vi "medicaoIXV.vi"() -> ()   [LabVIEW 2012]
uses:
  <vilib>/Utility/file.llb/Write To Spreadsheet File (string).vi
  <vilib>/Utility/file.llb/Write To Spreadsheet File (DBL).vi
  <instrlib>/Agilent 6XXX Series/Agilent 6XXX Series.lvlib
panel:
  out "reset graph":bool=TRUE
  out "tabela":dbl[][](array[numeric])
  in  "Tab Control":enum32{"Entrada de dados", "Saída de dados"}(tab)
  in  "T.J":dbl caption="Tensão\ndo joelho"
  in  "p.a.j":dbl caption="Pontos antes\ndo joelho"
  in  "nMedições":i16=1 caption="N° medições" min=1
  in  "area":dbl caption="Área da célula"
  in  "Tipo":string caption="Tipo da célula"
  in  "Formato":u16(ring) items=[".txt", ".csv"]
  out "ON/OFF1":bool caption="ON/OFF"
  in  "p.d.j":dbl caption="Pontos depois\ndo joelho"
  in  "T.M":dbl caption="Tensão máxima"
  in  "Nome da célula":string
  in  "Local":path
  in  "Delay(ms)":dbl
  in  "Start":bool
  in  "temperatura":dbl caption="Temperatura da célula"
  in  "stopProgram":bool caption="Parar Programa"
  out "Imp":dbl
  out "Vmp":dbl
  out "Pmp":dbl
  out "Icc (A)":dbl
  out "Vca (V)":dbl
  in  "Print Screen":bool
  out "IXV":cluster{"Y":dbl[], "Y":dbl[]}[](graph)
  out "output voltage":dbl
  out "vAtual":dbl caption="Tensao Atual (V)"
  out "aAtual":dbl caption="Corrente Atual\n(A)"
  out "Ponto Atual":i32
  out "tabela":dbl[][](array[numeric]) caption="TABELA DE DADOS\nTensão(Fonte)      Pontos             Tensao           Corrente" format="%0.8f"
  in  "stop":bool caption="Parar Medição"
  out "ON/OFF2":bool caption="ON/OFF"
  in  "CorrenteGraph":dbl
  in  "TensaoGraph":dbl
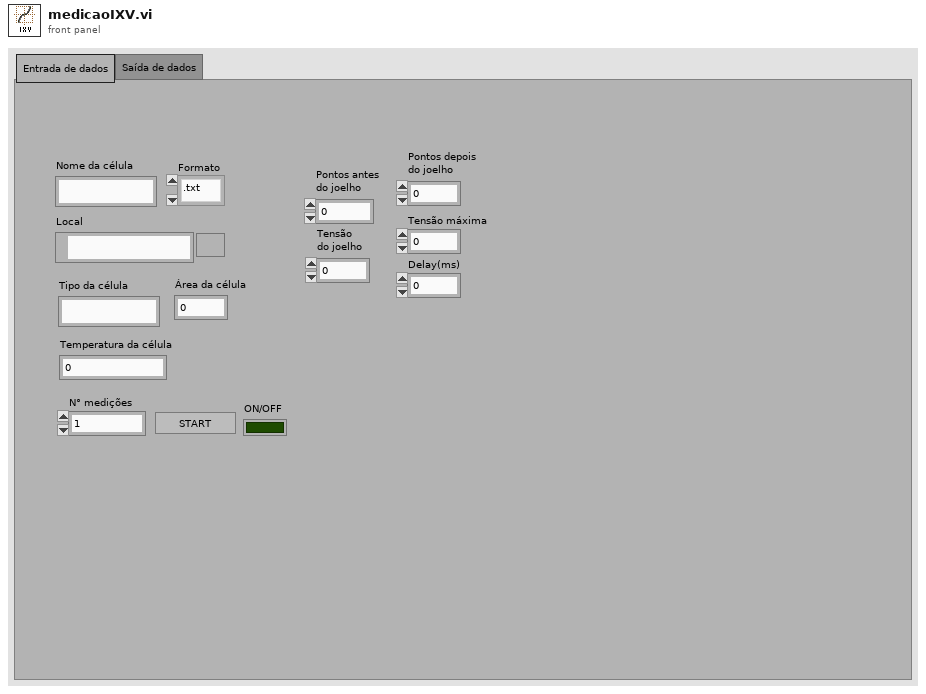
[diagram p1: front panel]
types:
  T1 = typedef "imagedata.ctl" = cluster{"image type":i32, "image depth":i32, "image":u8[], "mask":u8[], "colors":u32[], "Rectangle":cluster{"left":i16, "top":i16, "right":i16, "bottom":i16}}
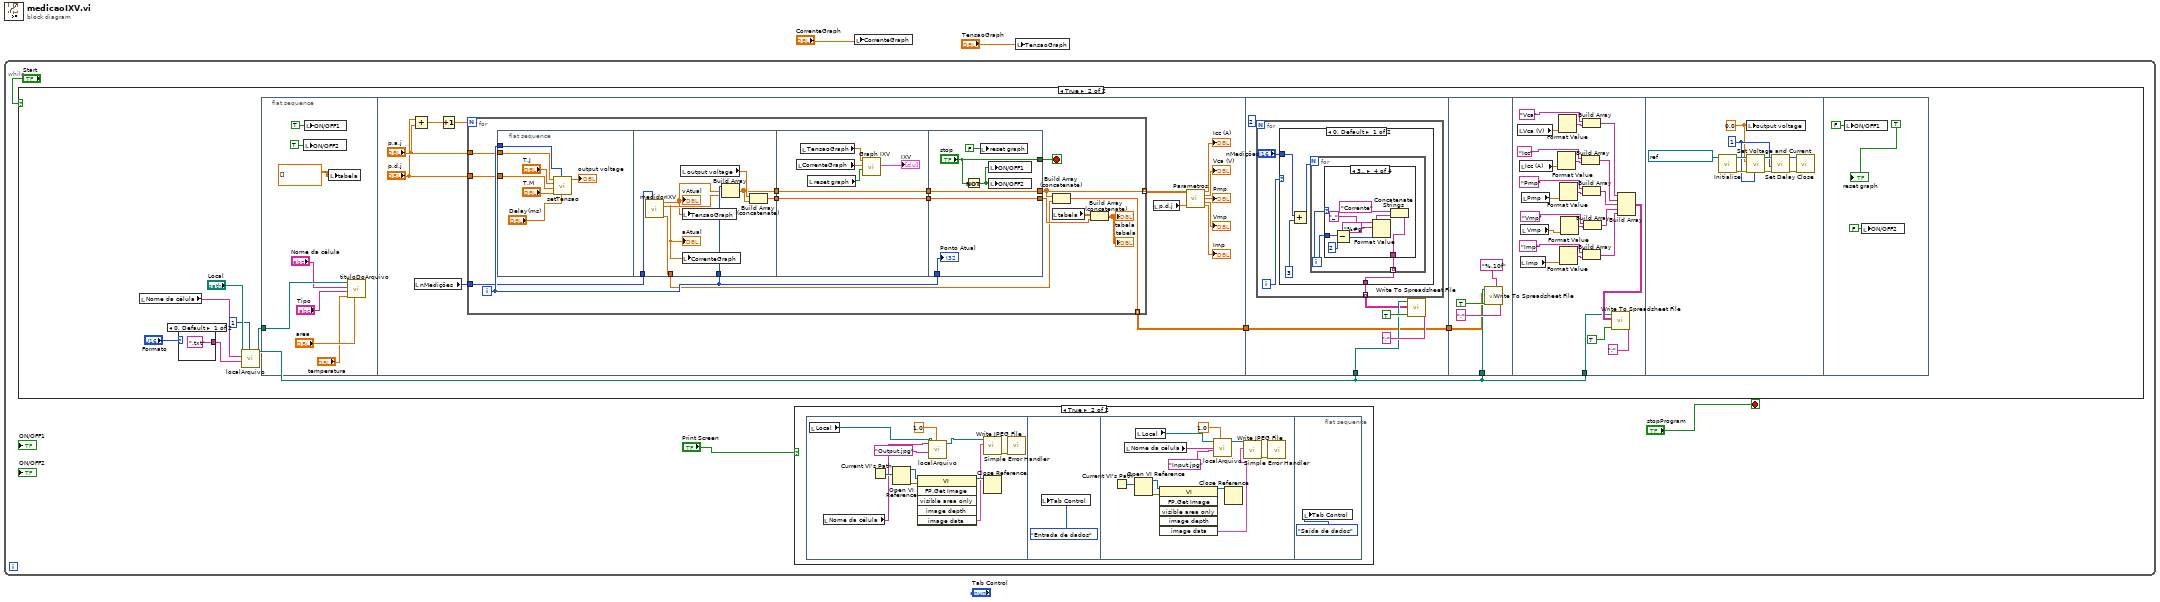
[diagram p0: block diagram]
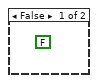
[diagram p3: hidden frame]
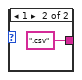
[diagram p4: hidden frame]
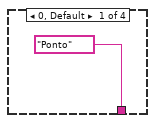
[diagram p5: hidden frame]
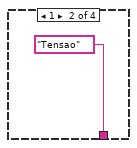
[diagram p6: hidden frame]
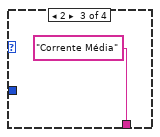
[diagram p7: hidden frame]
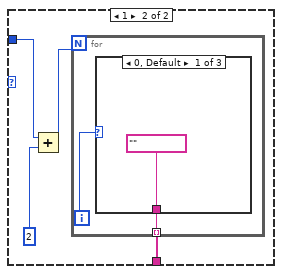
[diagram p8: hidden frame]
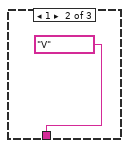
[diagram p9: hidden frame]
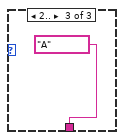
[diagram p10: hidden frame]
diagram:
  n1 = while {
    stop <- "stopProgram" stop-if-true
    n2 = case shown="True" "Start" {
      frame False {
        (unwired) FALSE
      }
      frame True {
        n3 = local read "Nome da célula"() -> (w35:string)
        n4 = case shown="0, Default" "Formato" {
          tunnel: [".txt" ".csv"] -> w34
          frame 0, Default {
          }
          frame 1 {
          }
        }
        n5 = call "localArquivo.vi"("quantidadeDeArquivos"=i16 1, "extensão"=w34, "Nome do arquivo"=w35, "Local"="Local") -> ("Path"=w33:path)  [unwired: 7 in]
        n6 = flat-sequence {
          tunnel: w33 -> [w47]
          tunnel: [w48] -> w30
          tunnel: w33 -> [w106]
          tunnel: [w103] -> w31
          tunnel: w30 -> [w103]
          tunnel: w33 -> [w139]
          tunnel: w31 -> [w138]
          tunnel: w33 -> [w143]
          frame #0 {
            n7 = local write "ON/OFF2"(TRUE ("ON/OFF2")) -> ()
            n8 = local write "ON/OFF1"(TRUE ("ON/OFF")) -> ()
            n9 = local write "tabela"(dbl[][] [] ("array")) -> ()
            n10 = call "tituloDoArquivo.vi"("area"="area", "temperatura"="temperatura", "Tipo"="Tipo", "Nome da célula"="Nome da célula", "file path (dialog if empty)"=w47) -> ()  [unwired: 7 in]
          }
          frame #1 {
            n11 = Add(x="p.d.j", y="p.a.j") -> (x+y=w53:dbl)
            n12 = local read "nMedições"() -> (w49:i16)
            n13 = Increment(x=w53) -> (x+1=w60:dbl)
            n14 = for {
              N: w60 -> [_]
              tunnel: [w63] -> w50 mode=indexing
              tunnel: "p.a.j" -> [w66]
              tunnel: "p.d.j" -> [w65]
              tunnel: w49 -> [w64]
              tunnel: [w61] -> w48 mode=indexing
              i -> [w70]
              stop <- w69 stop-if-true
              n15 = flat-sequence {
                tunnel: w70 -> [w81]
                tunnel: w66 -> [w79]
                tunnel: w65 -> [w78]
                tunnel: w70 -> [w87]
                tunnel: [w88] -> w75
                tunnel: [w90] -> w74
                tunnel: w64 -> [w84]
                tunnel: [w83] -> w62
                tunnel: [w96] -> w68
                tunnel: [w95] -> w67
                tunnel: w74 -> [w95]
                tunnel: w75 -> [w96]
                tunnel: [w101] -> w73
                tunnel: [w102] -> w63
                tunnel: w68 -> [w102]
                tunnel: w67 -> [w101]
                tunnel: w70 -> [w100]
                tunnel: ["stop"] -> w69
                frame #0 {
                  n16 = call "setTensao.vi"("delay(ms)"="Delay(ms)", "Ponto atual"=w81, "T.M"="T.M", "P.D.J"=w78, "T.J"="T.J", "P.A.J"=w79) -> ("output voltage"=→"output voltage":dbl)  [unwired: 5 in]
                }
                frame #1 {
                  n17 = call "medidorIXV.vi"("nMedicoes"=w84) -> ("Tensao Atual"=w85:dbl, "Corrente Atual"=w86:dbl, "vetorCorrente"=w83:dbl[])  [unwired: 7 in]
                  "aAtual" <- w86
                  "vAtual" <- w85
                  n18 = local read "output voltage"() -> (w89:dbl)
                  n19 = local write "TensaoGraph"(w85) -> ()
                  n20 = local write "CorrenteGraph"(w86) -> ()
                  n21 = Build Array(w87, w85, w86) -> (w88:dbl[])
                  n22 = Build Array (concatenate)(w89, w88) -> (w90:dbl[])
                }
                frame #2 {
                  n23 = local read "CorrenteGraph"() -> (w93:dbl)
                  n24 = local read "TensaoGraph"() -> (w94:dbl)
                  n25 = local read "reset graph"() -> (w91:bool)
                  n26 = call "Graph IXV"("Reset"=w91, "Y Input"=w93, "X Input"=w94) -> ("XY Graph"=→"IXV":cluster{"Y":dbl[], "Y":dbl[]}[])  [unwired: 2 in, 6 out]
                }
                frame #3 {
                  n27 = Not(x="stop") -> (.not. x?=w98:bool)
                  n28 = local write "reset graph"(FALSE) -> ()
                  n29 = local write "ON/OFF1"(w98) -> ()
                  n30 = local write "ON/OFF2"(w98) -> ()
                  "Ponto Atual" <- w100
                }
              }
              n31 = Build Array (concatenate)(w63, w62) -> (w61:dbl[])
              n32 = local read "tabela"() -> (w72:dbl[][])
              n33 = Build Array (concatenate)(w72, w73) -> (→"tabela" →"tabela":dbl[][])
            }
            n34 = local read "p.d.j"() -> (w59:dbl)
            n35 = call "Parametros.vi"("VetorDeDados"=w50, "pontos"=w59) -> ("Icc"=→"Icc (A)":dbl, "Vca"=→"Vca (V)":dbl, "Pmp"=→"Pmp":dbl, "Vmp"=→"Vmp":dbl, "Imp"=→"Imp":dbl)  [unwired: 9 in]
          }
          frame #2 {
            n36 = for {
              N: 2 -> [_]
              tunnel: [w109] -> w104 mode=indexing
              i -> [w111]
              n37 = case shown="0, Default" w111 {
                tunnel: "nMedições" -> [w113 w130]
                tunnel: [w112 w129] -> w109
                frame 0, Default {
                  n38 = Add(x=w113, y=i16 3) -> (x+y=w114:i16)
                  n39 = for {
                    N: w114 -> [_]
                    tunnel: [w116] -> w112 mode=indexing
                    i -> [w117]
                    n40 = case shown="3.." w117 {
                      tunnel: w117 -> [_ _ _ w125]
                      tunnel: ["Ponto" "Tensao" "Corrente Média" ("string") w123] -> w116
                      frame 0, Default {
                      }
                      frame 1 {
                      }
                      frame 2 {
                      }
                      frame 3.. {
                        n41 = Subtract(x=w125, y=2) -> (x-y=w126:i32)
                        n42 = Format Value(string ("")="_", format string="%#g", value (0)=w126) -> (output string=w127:string)
                        n43 = Concatenate Strings("Corrente" ("string"), w127) -> (w123:string)
                      }
                    }
                  }
                }
                frame 1 {
                  n44 = Add(x=w130, y=i16 2) -> (x+y=w131:i16)
                  n45 = for {
                    N: w131 -> [_]
                    tunnel: [w133] -> w129 mode=indexing
                    i -> [w134]
                    n46 = case shown="0, Default" w134 {
                      tunnel: ["" "V" "A" ("string")] -> w133
                      frame 0, Default {
                      }
                      frame 1 {
                      }
                      frame 2.. {
                      }
                    }
                  }
                }
              }
            }
            n47 = call-poly <vilib>:"Write To Spreadsheet File.vi"("delimiter (\\t)"=";" ("delimiter (\\t)"), "append to file? (new file:F)"=TRUE, "2D data"=w104, "file path (dialog if empty)"=w106) -> ()  [unwired: 4 in, 1 out]
          }
          frame #3 {
            n48 = call-poly <vilib>:"Write To Spreadsheet File.vi"("delimiter (\\t)"=";" ("delimiter (\\t)"), "format (%.3f)"="%.10f", "append to file? (new file:F)"=TRUE, "2D data"=w138, "file path (dialog if empty)"=w139) -> ()  [unwired: 3 in, 1 out]
          }
          frame #4 {
            n49 = local read "Vca (V)"() -> (w145:dbl)
            n50 = local read "Icc (A)"() -> (w155:dbl)
            n51 = local read "Imp"() -> (w158:dbl)
            n52 = local read "Vmp"() -> (w157:dbl)
            n53 = local read "Pmp"() -> (w156:dbl)
            n54 = Format Value(value (0)=w155) -> (output string=w148:string)  [unwired: 2 in]
            n55 = Format Value(value (0)=w145) -> (output string=w146:string)  [unwired: 2 in]
            n56 = Format Value(value (0)=w156) -> (output string=w150:string)  [unwired: 2 in]
            n57 = Format Value(value (0)=w158) -> (output string=w154:string)  [unwired: 2 in]
            n58 = Format Value(value (0)=w157) -> (output string=w152:string)  [unwired: 2 in]
            n59 = Build Array("Icc", w148) -> (w160:string[])
            n60 = Build Array("Vca", w146) -> (w159:string[])
            n61 = Build Array("Pmp", w150) -> (w161:string[])
            n62 = Build Array("Imp", w154) -> (w163:string[])
            n63 = Build Array("Vmp", w152) -> (w162:string[])
            n64 = Build Array(w159, w160, w161, w162, w163) -> (w164:string[][])
            n65 = call-poly <vilib>:"Write To Spreadsheet File.vi"("delimiter (\\t)"=";" ("delimiter (\\t)"), "append to file? (new file:F)"=TRUE, "2D data"=w164, "file path (dialog if empty)"=w143) -> ()  [unwired: 4 in, 1 out]
          }
          frame #5 {
            w167 = 0.0 ("voltage (0 V)")
            w170 = u8 1 ("channel (1)")
            n66 = call <instrlib>:"Initialize.vi"("VISA resource name"=refnum<visa-resource-name> "GPIB0::5::INSTR") -> ("error out"=w172:errorcluster, "VISA resource name out"=w171:refnum<visa-resource-name>)  [unwired: 9 in]
            n67 = local write "output voltage"(w167) -> ()
            n68 = call <instrlib>:"Set Voltage and Current.vi"("channel (1)"=w170, "error in (no error)"=w172, "voltage (0 V)"=w167, "VISA resource name"=w171) -> ("error out"=w173:errorcluster, "VISA resource name out"=w174:refnum<visa-resource-name>)  [unwired: 6 in]
            n69 = call <instrlib>:"Set Delay.vi"("error in (no error)"=w173, "channel (1)"=w170, "VISA resource name"=w174) -> ("error out"=w168:errorcluster, "VISA resource name out"=w169:refnum<visa-resource-name>)  [unwired: 7 in]
            n70 = call <instrlib>:"Close.vi"("error in (no error)"=w168, "VISA resource name"=w169) -> ()  [unwired: 9 in, 1 out]
          }
          frame #6 {
            n71 = local write "ON/OFF1"(FALSE) -> ()
            n72 = local write "ON/OFF2"(FALSE ("ON/OFF")) -> ()
            "reset graph" <- TRUE
          }
        }
      }
    }
    n73 = case shown="True" "Print Screen" {
      frame False {
      }
      frame True {
        n74 = flat-sequence {
          frame #0 {
            n75 = local read "Local"() -> (w9:path)
            n76 = local read "Nome da célula"() -> (w7:string)
            n77 = Current VI's Path() -> (path=w14:path)
            n78 = Open VI Reference(vi path=w14) -> (vi reference=w15:refnum<vi>, error out=w16:errorcluster)  [unwired: 5 in]
            n79 = invoke class="VI" method="FP.Get Image"(reference=w15, error in=w16) -> (reference out=w13:refnum<vi>, "image data"=w12:T1)  [unwired: 4 in, 4 out]
            n80 = call "localArquivo.vi"("quantidadeDeArquivos"=1.0, "extensão"="Output.jpg", "Nome do arquivo"=w7, "Local"=w9) -> ("Path"=w6:path)  [unwired: 7 in]
            n81 = call <vilib>:"Write JPEG File.vi"("image data"=w12, "path to JPEG file"=w6) -> ("error out"=w11:errorcluster)  [unwired: 8 in, 1 out]
            n82 = Close Reference(reference=w13) -> ()  [unwired: 1 in, 1 out]
            n83 = call <vilib>:"Simple Error Handler.vi"("error in (no error)"=w11) -> ()  [unwired: 4 in, 5 out]
          }
          frame #1 {
            n84 = local write "Tab Control"(enum32{"Entrada de dados", "Saída de dados"}."Entrada de dados" ("Tab Control")) -> ()
          }
          frame #2 {
            n85 = Current VI's Path() -> (path=w27:path)
            n86 = local read "Nome da célula"() -> (w21:string)
            n87 = Open VI Reference(vi path=w27) -> (vi reference=w26:refnum<vi>, error out=w25:errorcluster)  [unwired: 5 in]
            n88 = local read "Local"() -> (w20:path)
            n89 = invoke class="VI" method="FP.Get Image"(reference=w26, error in=w25) -> (reference out=w28:refnum<vi>, "image data"=w23:T1)  [unwired: 4 in, 4 out]
            n90 = call "localArquivo.vi"("quantidadeDeArquivos"=1.0, "extensão"="Input.jpg", "Nome do arquivo"=w21, "Local"=w20) -> ("Path"=w19:path)  [unwired: 7 in]
            n91 = Close Reference(reference=w28) -> ()  [unwired: 1 in, 1 out]
            n92 = call <vilib>:"Write JPEG File.vi"("image data"=w23, "path to JPEG file"=w19) -> ("error out"=w24:errorcluster)  [unwired: 8 in, 1 out]
            n93 = call <vilib>:"Simple Error Handler.vi"("error in (no error)"=w24) -> ()  [unwired: 4 in, 5 out]
          }
          frame #3 {
            n94 = local write "Tab Control"(enum32{"Entrada de dados", "Saída de dados"}."Saída de dados" ("Tab Control")) -> ()
          }
        }
      }
    }
  }
  n95 = local write "CorrenteGraph"("CorrenteGraph") -> ()
  n96 = local write "TensaoGraph"("TensaoGraph") -> ()
